vi "Agilent 34401 Acquire and Chart - External Triggered.vi"() -> ()   [LabVIEW 2013]
doc: "This example shows how to configure an externally triggered measurement using the low-level Data VIs to retrieve data from the DMM.\n\n<B>Note:</B>\n\n(1) It is recommended that all triggered measurements be made using an appropriate fixed manual range. That is, disable autorange and manually select a range in <B>Configure Measurement VI</B>.\n\n(2) To increase the speed of DC measurements, set Autozero to \"once,\" or \"off\" in <B>Configure Autozero VI</B>. \n\n(3) For faster AC measurements, call the Configure AC Filter VI to set the AC filter to 200 Hz, and set the manual trigger delay to 0 seconds in <B>Configure Trigger VI</B>."
uses:
  <vilib>/Utility/error.llb/DialogType.ctl
  <instrlib>/Agilent 34401/Agilent 34401.lvlib
panel:
  in  "Timeout (10000 ms)":u32=10000
  out "Measurements":dbl[](graph)
  in  "Slope (0: Negative)":u16(ring) items=["Negative", "Positive"]
  in  "Stop":bool
  in  "Manual Range (1.00)":dbl=1.0 format="%_3f"
  in  "Enable Auto Range (F: Disable)":bool
  in  "Function (0: DC Voltage)":u16(ring) items=["DC Voltage", "AC Voltage", "2 - Wire Resistance", "4 - Wire Resistance", "DC Current", "AC Current", "Frequency", "Period", "Continuity", "Diode Checking", "VDC:VDC Ratio", "Temperature", "Capacitance"]
  in  "Manual Trigger Delay (0.0 s)":dbl format="%.3f"
  in  "Enable Auto Delay (T: Enable)":bool=TRUE
  in  "Samples per Trigger (10)":i32=10 format="%#.6g"
  in  "Trigger Count (5)":i32=5 format="%#.6g"
  in  "VISA resource name":refnum<visa-resource-name>
  # "(c) 2005-2008 National Instruments.  ALL RIGHTS RESERVED."
  # "Note: This example requires an external trigger connected to the instrument!"
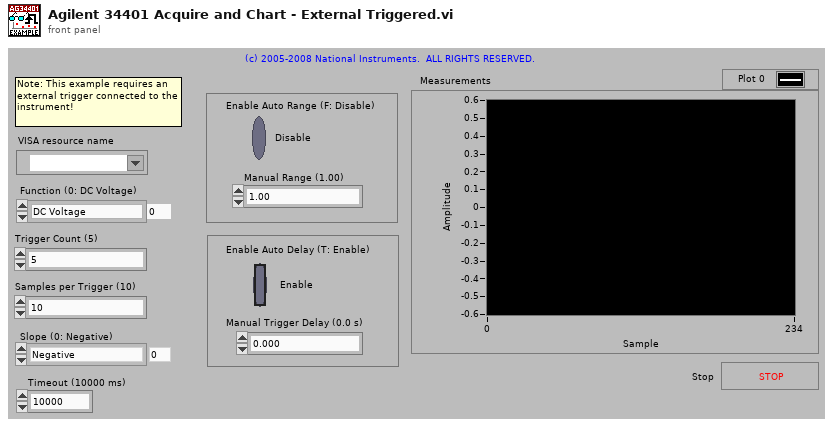
[diagram p1: front panel]
types:
  T1 = typedef "DialogType.ctl" = u16
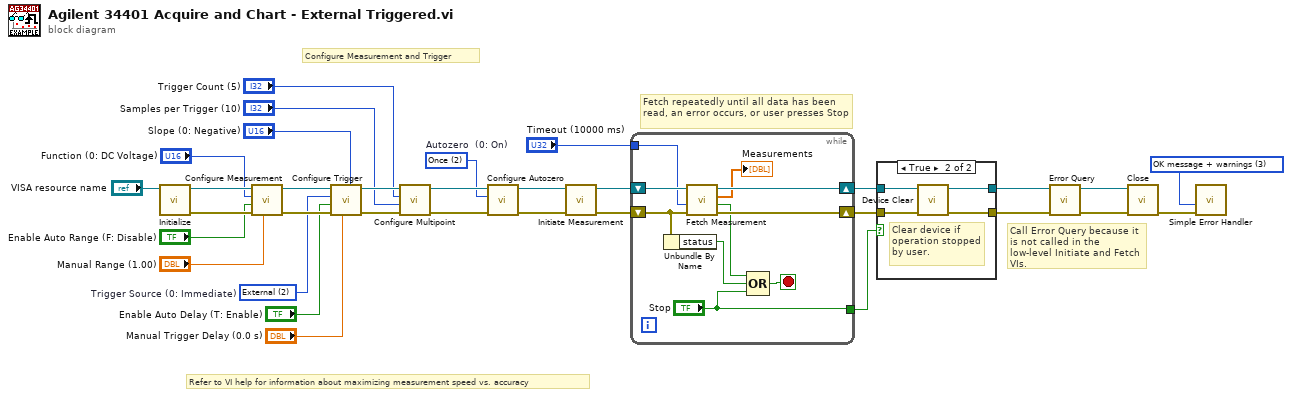
[diagram p0: block diagram]
diagram:
  w12 = T1 3 items=["no dialog", "OK message", "continue or stop message", "OK message + warnings", "continue/stop + warnings"] ("type of dialog (OK msg:1)")
  w20 = u16 2 items=["Immediate", "Software (Bus)", "External"]  # Trigger Source (0: Immediate)
  w23 = u16 2 items=["On", "Off", "Once"]  # Autozero  (0: On)
  # "Call Error Query because it is not called in the low-level Initiate and Fetch VIs."
  # "Fetch repeatedly until all data has been read, an error occurs, or user presses Stop"
  # "Refer to VI help for information about maximizing measurement speed vs. accuracy"
  # "Configure Measurement and Trigger"
  n1 = call <instrlib>:"Initialize.vi"("VISA resource name"="VISA resource name") -> ("error out"=w31:errorcluster, "VISA resource name out"=w32:refnum<visa-resource-name>)  [unwired: 9 in]
  n2 = call <instrlib>:"Configure Measurement.vi"("Manual Range (1.00)"="Manual Range (1.00)", "error in (no error)"=w31, "Enable Auto Range (T: Enable)"="Enable Auto Range (F: Disable)", "Function (0: DC Voltage)"="Function (0: DC Voltage)", "VISA resource name"=w32) -> ("error out"=w29:errorcluster, "VISA resource name out"=w30:refnum<visa-resource-name>)  [unwired: 5 in]
  n3 = call <instrlib>:"Configure Trigger.vi"("Slope (0: Negative)"="Slope (0: Negative)", "Manual Trigger Delay (0.0 s)"="Manual Trigger Delay (0.0 s)", "error in (no error)"=w29, "Enable Auto Delay (T: Enable)"="Enable Auto Delay (T: Enable)", "Trigger Source (0: Immediate)"=w20, "VISA resource name"=w30) -> ("error out"=w27:errorcluster, "VISA resource name out"=w28:refnum<visa-resource-name>)  [unwired: 4 in]
  n4 = call <instrlib>:"Configure Multipoint.vi"("error in (no error)"=w27, "Sample Count (1)"="Samples per Trigger (10)", "Trigger Count (1)"="Trigger Count (5)", "VISA resource name"=w28) -> ("error out"=w25:errorcluster, "VISA resource name out"=w24:refnum<visa-resource-name>)  [unwired: 6 in]
  n5 = call <instrlib>:"Configure Autozero.vi"("error in (no error)"=w25, "Autozero  (0: On)"=w23, "VISA resource name"=w24) -> ("error out"=w22:errorcluster, "VISA resource name out"=w21:refnum<visa-resource-name>)  [unwired: 7 in]
  n6 = call <instrlib>:"Initiate Measurement.vi"("error in (no error)"=w22, "VISA resource name"=w21) -> ("error out"=w11:errorcluster, "VISA resource name out"=w10:refnum<visa-resource-name>)  [unwired: 8 in]
  n7 = while {
    tunnel: ["Stop"] -> w6
    shift-right: [w43] -> w7
    shift-left: w10 -> [w41]
    shift-right: [w42] -> w8
    shift-left: w11 -> [w37]
    tunnel: "Timeout (10000 ms)" -> [w34]
    stop <- w39 stop-if-true
    n8 = Unbundle By Name(w37) -> ("status"=w36:bool)
    n9 = call <instrlib>:"Fetch Measurement.vi"("error in (no error)"=w37, "Timeout (10000 ms)"=w34, "VISA resource name"=w41) -> ("error out"=w42:errorcluster, "End of Data?"=w40:bool, "Measurements"=→"Measurements":dbl[], "VISA resource name out"=w43:refnum<visa-resource-name>)  [unwired: 5 in]
    n10 = Compound Arithmetic op=OR(w40, w36, "Stop") -> (w39:bool)
  }
  n11 = case shown="True" w6 {
    tunnel: w8 -> [w44 w49]
    tunnel: [w44 w46] -> w2
    tunnel: w7 -> [w45 w48]
    tunnel: [w45 w47] -> w3
    frame False {
    }
    frame True {
      # "Clear device if operation stopped by user."
      n12 = call <instrlib>:"Device Clear.vi"("error in (no error)"=w49, "VISA Resource Name"=w48) -> ("error out"=w46:errorcluster, "VISA Resource Out"=w47:refnum<visa-resource-name>)  [unwired: 8 in]
    }
  }
  n13 = call <instrlib>:"Error Query.vi"("error in (no error)"=w2, "VISA resource name"=w3) -> ("error out"=w5:errorcluster, "VISA resource name out"=w4:refnum<visa-resource-name>)  [unwired: 6 in, 2 out]
  n14 = call <instrlib>:"Close.vi"("error in (no error)"=w5, "VISA resource name"=w4) -> ("error out"=w26:errorcluster)  [unwired: 9 in]
  n15 = call <vilib>:"Simple Error Handler.vi"("type of dialog (OK msg:1)"=w12, "error in (no error)"=w26) -> ()  [unwired: 3 in, 5 out]
